vi "Dhoot Top Coordinate System 2.vi"(0 "Image Out":T8(plugin-control), 1 "Edge Options ROI 1":T5={"Edge Polarity"=0, "Kernel Size"=3, "Width"=3, "Minimum Edge Strength"=10.0, "Interpolation Type"=enum."Bilinear Fixed", "Data Processing Method"=enum."Average"} {"Edge Polarity" items=["All Edges", "Rising Edges", "Falling Edges"]; "Minimum Edge Strength" format="%.2f"; "Width" step=2; "Kernel Size" step=2}, 2 "Edge Options ROI 2":T5={"Edge Polarity"=0, "Kernel Size"=3, "Width"=3, "Minimum Edge Strength"=10.0, "Interpolation Type"=enum."Bilinear Fixed", "Data Processing Method"=enum."Average"} {"Edge Polarity" items=["All Edges", "Rising Edges", "Falling Edges"]; "Minimum Edge Strength" format="%.2f"; "Width" step=2; "Kernel Size" step=2}, 3 "Line Options ROI 1":T3={"Number of Lines"=1, "Type"=enum."First Edge Rake", "Min. Score"=10.0, "Max. Score"=1000.0, "Orientation"=0.0, "Angle Range"=45.0, "Angle Tolerance"=1.0, "Step Size"=7, "Min. SNR (db)"=0.0, "Min. Points (%)"=25.0, "Hough Iterations"=5} {"Min. Points (%)" min=0.0 max=100.0; "Min. SNR (db)" min=0.0; "Max. Score" min=0.0 max=1024.0; "Min. Score" min=0.0 max=1024.0 step=1.0}, 4 "Line Options ROI 2":T3={"Number of Lines"=1, "Type"=enum."First Edge Rake", "Min. Score"=10.0, "Max. Score"=1000.0, "Orientation"=0.0, "Angle Range"=45.0, "Angle Tolerance"=1.0, "Step Size"=7, "Min. SNR (db)"=0.0, "Min. Points (%)"=25.0, "Hough Iterations"=5} {"Min. Points (%)" min=0.0 max=100.0; "Min. SNR (db)" min=0.0; "Max. Score" min=0.0 max=1024.0; "Min. Score" min=0.0 max=1024.0 step=1.0}, 5 "error in (no error)":errorcluster, 6 "ROI 1":T2 {"Contours"."Type" items=["No Selection", "Point", "Line", "Rectangle", "Oval", "Polygon", "Free", "Annulus", "Unused2", "Unused3", "Broken Line", "Free Hand Line", "Rotated Rectangle"]}, 7 "Search Direction ROI 1":u32, 8 "ROI 2":T2 {"Contours"."Type" items=["No Selection", "Point", "Line", "Rectangle", "Oval", "Polygon", "Free", "Annulus", "Unused2", "Unused3", "Broken Line", "Free Hand Line", "Rotated Rectangle"]}, 9 "Search Direction ROI 2":u32, 10 "OverlayOptions":T1) -> (14 "Co ordinate System":T7, 19 "error out":errorcluster)   [LabVIEW 2019, in "Algorithm.lvclass"]
uses:
  FrameworkOverrides/Algorithm.lvclass
  <vilib>/vision/NI_Vision_Development_Module.lvlib
  <vilib>/vision/Measure.llb/Edge Polarity.ctl
  <vilib>/vision/Measure.llb/Edge Options.ctl
  <vilib>/vision/Measure.llb/Straight Edge Process.ctl
  <vilib>/vision/Measure.llb/Straight Edge Options.ctl
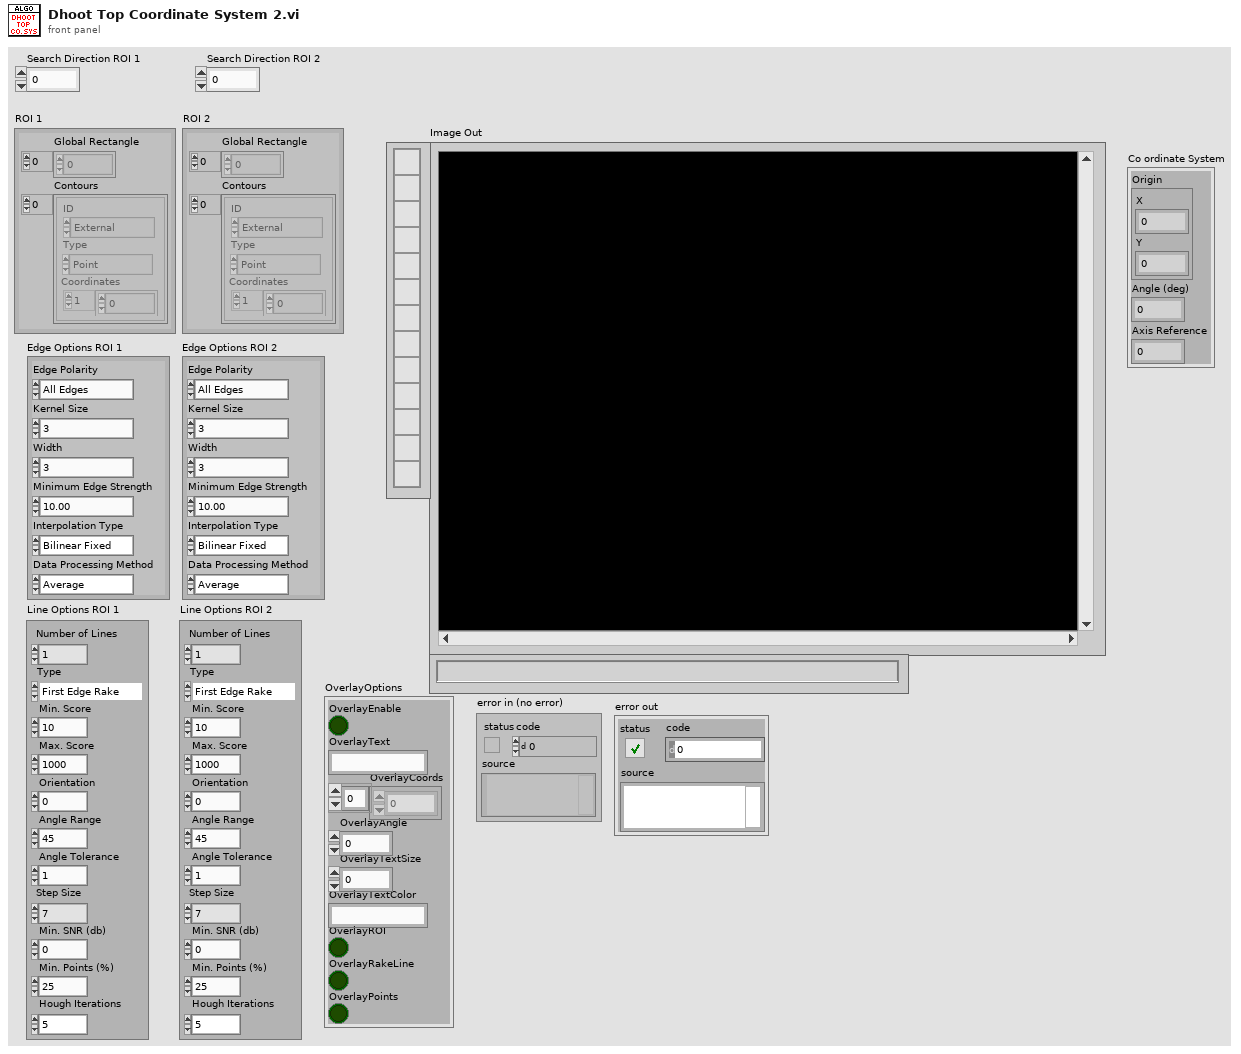
[diagram p1: front panel]
types:
  T1 = cluster{"OverlayEnable":bool, "OverlayText":string, "OverlayCoords":i32[], "OverlayAngle":i32, "OverlayTextSize":i32, "OverlayTextColor":string, "OverlayROI":bool, "OverlayRakeLine":bool, "OverlayPoints":bool}
  T2 = cluster{"Global Rectangle":i32[], "Contours":cluster{"ID":enum32{"External", "Internal"}, "Type":u32, "Coordinates":i32[]}[]}
  T3 = typedef "Straight Edge Options.ctl" = cluster{"Number of Lines":i32, "Type":T4, "Min. Score":dbl, "Max. Score":dbl, "Orientation":dbl, "Angle Range":dbl, "Angle Tolerance":dbl, "Step Size":u32, "Min. SNR (db)":dbl, "Min. Points (%)":dbl, "Hough Iterations":i32}
  T4 = typedef "Straight Edge Process.ctl" = enum32{"First Edge Rake", "Best Edge Rake", "Hough Edge Rake", "First Edge Projection", "Best Edge Projection"}
  T5 = typedef "Edge Options.ctl" = cluster{"Edge Polarity":T6, "Kernel Size":u32, "Width":u32, "Minimum Edge Strength":sgl, "Interpolation Type":enum32{"Zero Order", "Bilinear", "Quadratic", "Cubic", "Bilinear Fixed"}, "Data Processing Method":enum32{"Average", "Median"}}
  T6 = typedef "Edge Polarity.ctl" = u32
  T7 = cluster{"Origin":cluster{"X":sgl, "Y":sgl}, "Angle (deg)":sgl, "Axis Reference":u32}
  T8 = typedef "IMAQ Image.ctl" = refnum<image>
  T9 = typedef "IMAQ Rectangle" = cluster{"Left":i32, "Top":i32, "Right":i32, "Bottom":i32, "Rotation":dbl}
  T10 = cluster{"Search Direction":u32, "Edge Options":T5, "Show Search Area":bool, "Show Search Lines":bool, "Show Edges Found":bool, "Show Result":bool, "Search Area Color":u32, "Search Lines Color":u32, "Edge Locations Color":u32, "Result Color":u32, "Overlay Group Name":string}
  T11 = cluster{"Point1 (Pixels)":cluster{"X":sgl, "Y":sgl}, "Point2 (Pixels)":cluster{"X":sgl, "Y":sgl}, "Point1 (Real-World)":cluster{"X":sgl, "Y":sgl}, "Point2 (Real-World)":cluster{"X":sgl, "Y":sgl}, "Angle (Pixel)":dbl, "Angle (Real-World)":dbl, "Score":dbl, "Straightness":dbl, "Average SNR (db)":dbl, "Calibration Valid":bool}[]
  T12 = cluster{"Point1 (Pixels)":cluster{"X":sgl, "Y":sgl}, "Point2 (Pixels)":cluster{"X":sgl, "Y":sgl}, "Point1 (Real-World)":cluster{"X":sgl, "Y":sgl}, "Point2 (Real-World)":cluster{"X":sgl, "Y":sgl}, "Angle (Pixel)":dbl, "Angle (Real-World)":dbl, "Score":dbl, "Straightness":dbl, "Average SNR (db)":dbl, "Calibration Valid":bool}
  T13 = cluster{"Point1 (Pixels)":cluster{"X":sgl, "Y":sgl}, "Point2 (Pixels)":cluster{"X":sgl, "Y":sgl}}
  T14 = typedef "ROI Descriptor" = cluster{"Global Rectangle":i32[], "Contours":cluster{"ID":enum32{"External", "Internal"}, "Type":u32, "Coordinates":i32[]}[]}
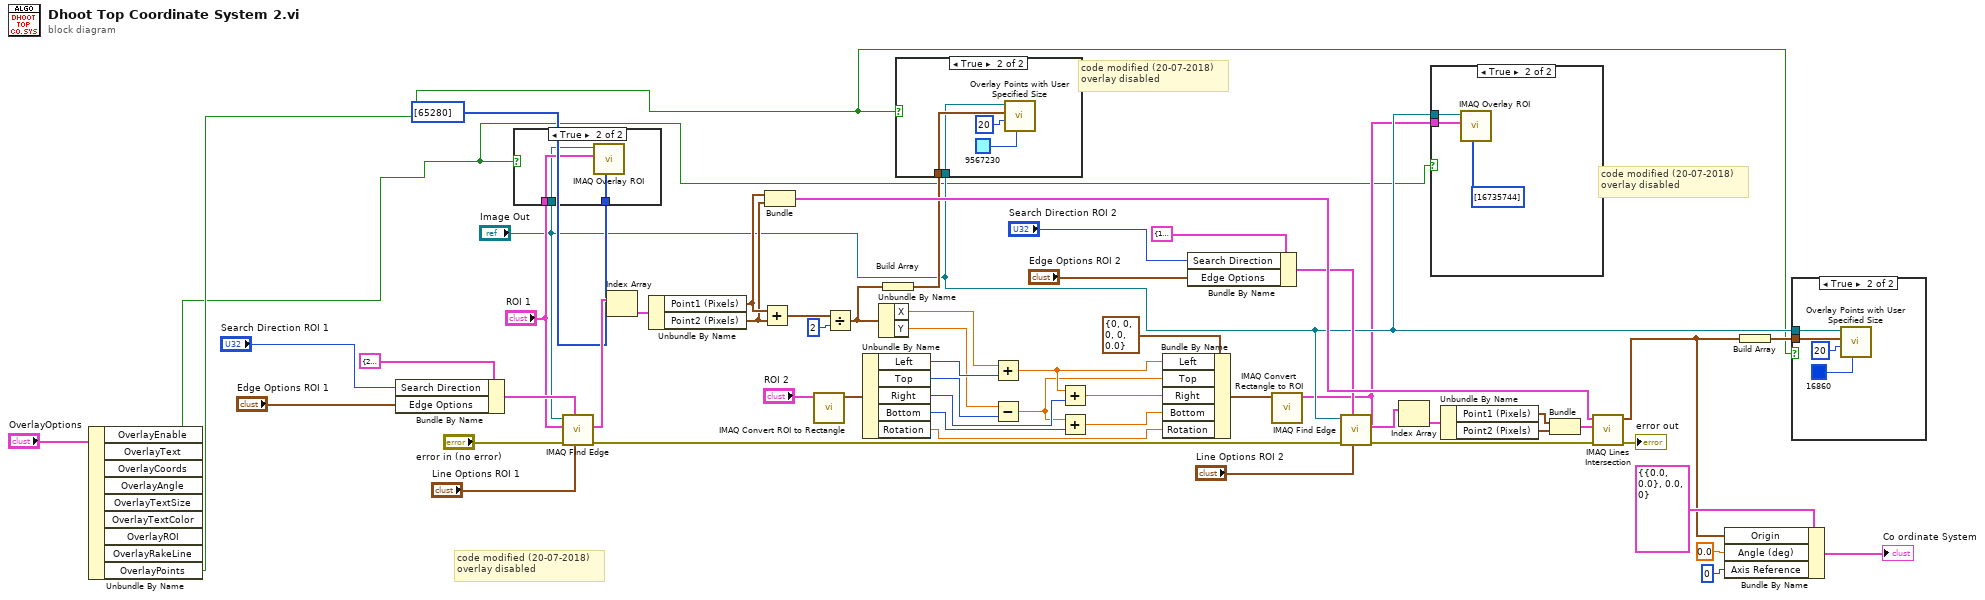
[diagram p0: block diagram]
diagram:
  # "code modified (20-07-2018)\noverlay disabled"
  # "code modified (20-07-2018)\noverlay disabled"
  # "code modified (20-07-2018)\noverlay disabled"
  n1 = Unbundle By Name("OverlayOptions") -> ("OverlayROI"=w1:bool, "OverlayPoints"=w2:bool)  [unwired: 7 out]
  n2 = Bundle By Name(cluster=T10 {"Search Direction"=2, "Edge Options"={"Edge Polarity"=0, "Kernel Size"=5, "Width"=5, "Minimum Edge Strength"=50.0, "Interpolation Type"=enum."Bilinear Fixed", "Data Processing Method"=enum."Average"}, "Show Search Area"=FALSE, "Show Search Lines"=FALSE, "Show Edges Found"=FALSE, "Show Result"=TRUE, "Search Area Color"=65280, "Search Lines Color"=255, "Edge Locations Color"=16776960, "Result Color"=16711680, "Overlay Group Name"=""} ("Options"), "Search Direction"="Search Direction ROI 1", "Edge Options"="Edge Options ROI 1") -> (w37:T10)
  n3 = case shown="True" w1 {
    tunnel: "ROI 1" -> [_ w59]
    tunnel: u32[] [65280] ("Colors (Green)") -> [_ w58]
    tunnel: "Image Out" -> [_ w57]
    frame False {
    }
    frame True {
      n4 = call "IMAQ Overlay ROI"("Colors (Green)"=w58, "ROI Descriptor"=w59, "Image"=w57) -> ()  [unwired: 7 in, 2 out]
    }
  }
  n5 = call "IMAQ Find Edge"("Line Fit Options"="Line Options ROI 1", "Options"=w37, "error in (no error)"="error in (no error)", "ROI Descriptor"="ROI 1", "Image"="Image Out") -> ("error out"=w26:errorcluster, "Straight Edges"=w54:T11)  [unwired: 3 in, 2 out]
  n6 = Index Array(array=w54) -> (element=w52:T12)  [unwired: 1 in]
  n7 = Unbundle By Name(w52) -> ("Point1 (Pixels)"=w24:cluster{"X":sgl, "Y":sgl}, "Point2 (Pixels)"=w23:cluster{"X":sgl, "Y":sgl})
  n8 = Add(x=w24, y=w23) -> (x+y=w22:cluster{"X":sgl, "Y":sgl})
  n9 = Bundle("Point1 (Pixels)"=w24, "Point2 (Pixels)"=w23) -> (w50:T13)  [unwired: 1 in]
  n10 = call "IMAQ Convert ROI to Rectangle"("ROI Descriptor"="ROI 2") -> ("Rectangle"=w27:T9)  [unwired: 8 in, 1 out]
  n11 = Divide(x=w22, y=2) -> (x/y=w17:cluster{"X":sgl, "Y":sgl})
  n12 = Unbundle By Name(w27) -> ("Left"=w15:i32, "Top"=w9:i32, "Right"=w12:i32, "Bottom"=w8:i32, "Rotation"=w19:dbl)
  n13 = Unbundle By Name(w17) -> ("X"=w14:sgl, "Y"=w10:sgl)
  n14 = Build Array(w17) -> (w18:cluster{"X":sgl, "Y":sgl}[])
  n15 = case shown="True" w2 {
    tunnel: w18 -> [_ w61]
    tunnel: "Image Out" -> [_ w60]
    frame False {
    }
    frame True {
      n16 = call "Overlay Points with User Specified Size.vi"("Color"=u32 9567230, "Point Diameter (5)"=u32 20, "Points"=w61, "Image In"=w60) -> ()  [unwired: 6 in, 2 out]
    }
  }
  n17 = Add(x=w14, y=w15) -> (x+y=w13:sgl)
  n18 = Subtract(x=w10, y=w9) -> (x-y=w6:sgl)
  n19 = Add(x=w13, y=w12) -> (x+y=w11:sgl)
  n20 = Add(x=w6, y=w8) -> (x+y=w7:sgl)
  n21 = Bundle By Name(cluster=T9 {"Left"=0, "Top"=0, "Right"=0, "Bottom"=0, "Rotation"=0.0} ("Rectangle"), "Left"=w13, "Top"=w6, "Right"=w11, "Bottom"=w7, "Rotation"=w19) -> (w5:T9)
  n22 = Bundle By Name(cluster=T10 {"Search Direction"=1, "Edge Options"={"Edge Polarity"=0, "Kernel Size"=5, "Width"=5, "Minimum Edge Strength"=50.0, "Interpolation Type"=enum."Zero Order", "Data Processing Method"=enum."Average"}, "Show Search Area"=FALSE, "Show Search Lines"=FALSE, "Show Edges Found"=FALSE, "Show Result"=TRUE, "Search Area Color"=65280, "Search Lines Color"=255, "Edge Locations Color"=16776960, "Result Color"=16711680, "Overlay Group Name"=""} ("Options"), "Search Direction"="Search Direction ROI 2", "Edge Options"="Edge Options ROI 2") -> (w33:T10)
  n23 = call "IMAQ Convert Rectangle to ROI"("Rectangle"=w5) -> ("ROI Descriptor"=w4:T14)  [unwired: 8 in, 1 out]
  n24 = call "IMAQ Find Edge"("Line Fit Options"="Line Options ROI 2", "Options"=w33, "error in (no error)"=w26, "ROI Descriptor"=w4, "Image"="Image Out") -> ("error out"=w25:errorcluster, "Straight Edges"=w53:T11)  [unwired: 3 in, 2 out]
  n25 = Index Array(array=w53) -> (element=w51:T12)  [unwired: 1 in]
  n26 = case shown="True" w1 {
    tunnel: "Image Out" -> [_ w65]
    tunnel: w4 -> [_ w64]
    frame False {
    }
    frame True {
      n27 = call "IMAQ Overlay ROI"("Colors (Green)"=u32[] [16735744], "ROI Descriptor"=w64, "Image"=w65) -> ()  [unwired: 7 in, 2 out]
    }
  }
  n28 = Unbundle By Name(w51) -> ("Point1 (Pixels)"=w49:cluster{"X":sgl, "Y":sgl}, "Point2 (Pixels)"=w48:cluster{"X":sgl, "Y":sgl})
  n29 = Bundle("Point1 (Pixels)"=w49, "Point2 (Pixels)"=w48) -> (w47:T13)  [unwired: 1 in]
  n30 = call "IMAQ Lines Intersection"("error in (no error)"=w25, "Line 2"=w47, "Line 1"=w50) -> ("error out"=→"error out":errorcluster, "Intersection Point"=w42:cluster{"X":sgl, "Y":sgl})  [unwired: 6 in, 1 out]
  n31 = Bundle By Name(cluster=T7 {"Origin"={"X"=0.0, "Y"=0.0}, "Angle (deg)"=0.0, "Axis Reference"=0} ("Coordinate System"), "Origin"=w42, "Angle (deg)"=sgl 0.0, "Axis Reference"=u32 0) -> (→"Co ordinate System":T7)
  n32 = Build Array(w42) -> (w41:cluster{"X":sgl, "Y":sgl}[])
  n33 = case shown="True" w2 {
    tunnel: w41 -> [_ w70]
    tunnel: "Image Out" -> [_ w67]
    frame False {
    }
    frame True {
      n34 = call "Overlay Points with User Specified Size.vi"("Color"=u32 16860, "Point Diameter (5)"=u32 20, "Points"=w70, "Image In"=w67) -> ()  [unwired: 6 in, 2 out]
    }
  }
